vi "Read Conversion 2s Complement.vi"(9 "Input Read Data":u16) -> (3 "Coversion Output Data":dbl)   [LabVIEW 2023, in "HardwareAbstractionLayer_LVOOP.lvlib" / "Modbus.lvclass"]
uses:
  Modbus.lvclass
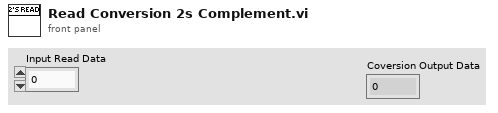
[diagram p1: front panel]
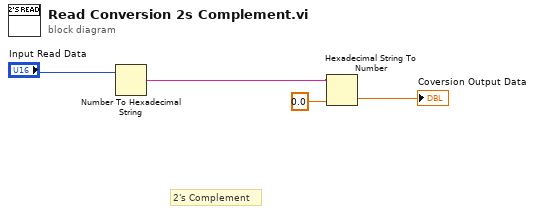
[diagram p0: block diagram]
diagram:
  # "2's Complement"
  n1 = Number To Hexadecimal String(2:"Input Read Data") -> (0:w3:string)  [unwired: 1 in]
  n2 = Hexadecimal String To Number(string=w3, default (0uL)=0.0) -> (number=→"Coversion Output Data":dbl)  [unwired: 1 in, 1 out]
